vi "Add Method.vi"(8 "error in (no error)":errorcluster, 10 "Method":refnum<class "Method.lvclass">, 11 "Class in":refnum<class "Class.lvclass">) -> (0 "error out":errorcluster, 3 "Class out":refnum<class "Class.lvclass">)   [LabVIEW 2017, in "Cobertura.lvlib" / "Class.lvclass"]
uses:
  Class.lvclass
  Method/Method.lvclass
  Class.lvclass/Class.ctl
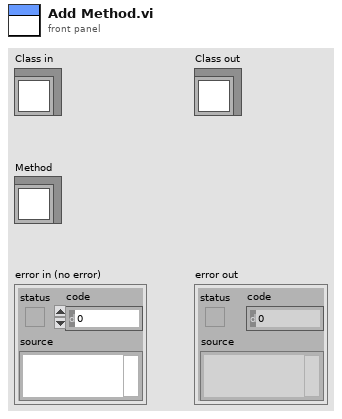
[diagram p1: front panel]
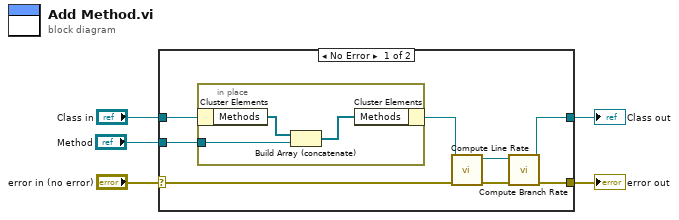
[diagram p0: block diagram]
diagram:
  n1 = case shown="No Error" "error in (no error)" {
    selector: "error in (no error)" -> [w10 w18]
    tunnel: [w8 w18] -> w4
    tunnel: [w7 w17] -> w2
    tunnel: "Class in" -> [w13 w17]
    tunnel: "Method" -> [w12 _]
    frame No Error {
      n2 = in-place {
        in-place-border: w12 -> [w14]
        n3 = in-place-cluster #1(w13) -> ("Methods"=w16:refnum<class "Method.lvclass">[])
        n4 = Build Array (concatenate)(w16, w14) -> (w15:refnum<class "Method.lvclass">[])
        n5 = in-place-cluster #1("Methods"=w15) -> (w6:refnum<class "Class.lvclass">)
      }
      n6 = call "Compute Line Rate.vi"("error in (no error)"=w10, "Class in"=w6) -> ("error out"=w9:errorcluster, "Class out"=w11:refnum<class "Class.lvclass">)  [unwired: 8 in]
      n7 = call "Compute Branch Rate.vi"("error in (no error)"=w9, "Class in"=w11) -> ("error out"=w8:errorcluster, "Class out"=w7:refnum<class "Class.lvclass">)  [unwired: 8 in]
    }
    frame Error {
    }
  }
  "error out" <- w4
  "Class out" <- w2
